vi "UR3_FK.vi"(11 "qs (deg)":sgl[](array[numeric])) -> (2 "end effector pose":T1=[[-0.17342125161384786, -0.98484285048279, 0.0031031180478863496, -0.3889317595458636], [0.9841770580893162, -0.17341855509434081, -0.03635275890011282, -0.2294631382444099], [0.03633989294625235, -0.003250323356801372, 0.9993342021459743, 0.4272266023792753], [0.0, 0.0, 0.0, 1.0]], 3 "3D Picture":refnum<vi>)   [LabVIEW 2024]
uses:
  <vilib>/Analysis/Matrix/Datatypes/RealMatrix.ctl
  <vilib>/Analysis/Matrix/NI_Matrix.lvlib
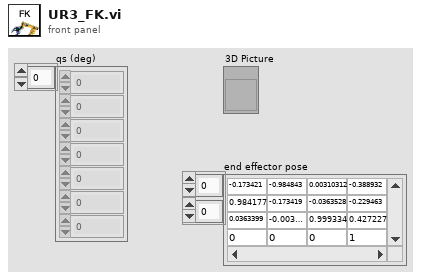
[diagram p1: front panel]
types:
  T1 = typedef "NI_Matrix.lvlib/RealMatrix.ctl" = dbl[][]
  T2 = cluster{"theta (deg)":dbl, "d":dbl, "a":dbl, "alpha (deg)":dbl}[]
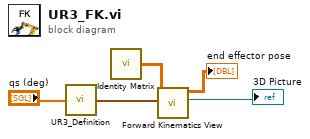
[diagram p0: block diagram]
diagram:
  n1 = call <userlib>:"UR3_Definition.vi"("qs (deg)"="qs (deg)") -> ("UR3"=w1:T2)
  n2 = call <userlib>:"Identity Matrix.vi"() -> ("Identity Matrix"=w4:T1)  [unwired: 1 in]
  n3 = call <userlib>:"Forward Kinematics View.vi"("Joints"=w1, "start pose"=w4) -> ("3D Picture"=→"3D Picture":refnum<vi>, "end effector pose"=→"end effector pose":T1)  [unwired: 8 in]
